vi "config_class.vi"(7 "config in":T1, 8 "error in (no error)":errorcluster, 11 "lv-builder in":refnum<class "lv-builder.lvclass">) -> (0 "error out":errorcluster, 3 "lv-builder out":refnum<class "lv-builder.lvclass">)   [LabVIEW 2015, in "lv-build-interface.lvlib"]
uses:
  lv-build-interface.lvlib
  lv-builder/class/lv-builder.lvclass
  lv-build/public/_controls/configuration.ctl
  lv-build/lv-build.lvlib
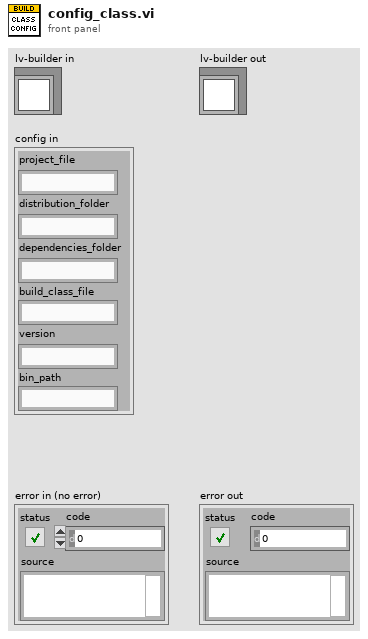
[diagram p1: front panel]
types:
  T1 = typedef "lv-build.lvlib/configuration.ctl" = cluster{"project_file":string, "distribution_folder":string, "dependencies_folder":string, "build_class_file":string, "version":string, "bin_path":string}
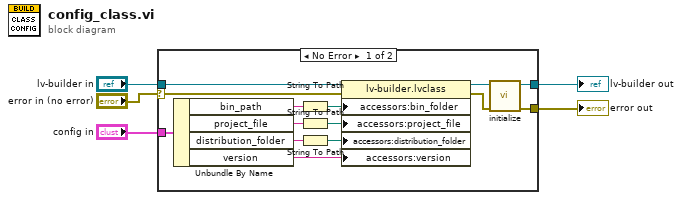
[diagram p0: block diagram]
diagram:
  n1 = case shown="No Error" "error in (no error)" {
    selector: "error in (no error)" -> [w18 w21]
    tunnel: [w6 w20] -> w5
    tunnel: [w7 w21] -> w4
    tunnel: "config in" -> [w19 _]
    tunnel: "lv-builder in" -> [w13 w20]
    frame No Error {
      n2 = Unbundle By Name(w19) -> ("bin_path"=w11:string, "project_file"=w12:string, "distribution_folder"=w14:string, "version"=w15:string)
      n3 = String To Path(string=w11) -> (path=w10:path)
      n4 = String To Path(string=w12) -> (path=w17:path)
      n5 = String To Path(string=w14) -> (path=w16:path)
      n6 = property class="lv-builder.lvclass"(reference=w13, error in=w18, "accessors:bin_folder"=w10, "accessors:project_file"=w17, "accessors:distribution_folder"=w16, "accessors:version"=w15) -> (reference out=w9:refnum<class "lv-builder.lvclass">, error out=w8:errorcluster)
      n7 = call-dynamic "initialize.vi"("error in (no error)"=w8, "lv-builder in"=w9) -> ("error out"=w7:errorcluster, "lv-builder out"=w6:refnum<class "lv-builder.lvclass">)  [unwired: 8 in]
    }
    frame Error {
    }
  }
  "lv-builder out" <- w5
  "error out" <- w4
